vi "Table.Clear.vi"(8 "error in (no error)":errorcluster, 11 "State Variables":T1) -> (0 "error out":errorcluster)   [LabVIEW 2015]
uses:
  Types/Main.StateVariables.ctl
  <vilib>/Utility/miscctls.llb/LVPositionTypeDef.ctl
  Types/Execute.UserEventRefs.ctl
  <vilib>/NI Veristand/Execution/Workspace/SystemStateRegEventRef.ctl
  <vilib>/NI Veristand/Execution/Workspace/Target State Info.ctl
  <vilib>/NI Veristand/Execution/Workspace/Target State.ctl
  <vilib>/NI Veristand/Execution/WaveformStreaming/Waveform Data Watcher Event Data (DBL).ctl
  <vilib>/NI Veristand/Execution/WaveformStreaming/WaveformStreamSpecification.ctl
  NationalInstruments.VeriStand.ClientAPI
  <vilib>/NI Veristand/Execution/Workspace/SystemStateEventRef.ctl
  <vilib>/NI Veristand/Execution/Workspace/WorkspaceAPI.ctl
  Types/UI.Object.ctl
  Types/Waveforms.Info.ctl
  <vilib>/NI Veristand/Execution/WaveformStreaming/Registered Waveform Streams Data Event Refnum (DBL).ctl
  <vilib>/NI Veristand/Execution/WaveformStreaming/WaveformDataWatcherDBL.ctl
  <vilib>/NI Veristand/Execution/WaveformStreaming/WaveformStreamingAPI.ctl
  <vilib>/Utility/miscctls.llb/LVRowAndColumnTypeDef.ctl
  <vilib>/NI Veristand/Execution/Workspace/NI_VS Workspace ExecutionAPI.lvlib
  <vilib>/NI Veristand/Execution/WaveformStreaming/NI_VS Waveform Streaming Interface.lvlib
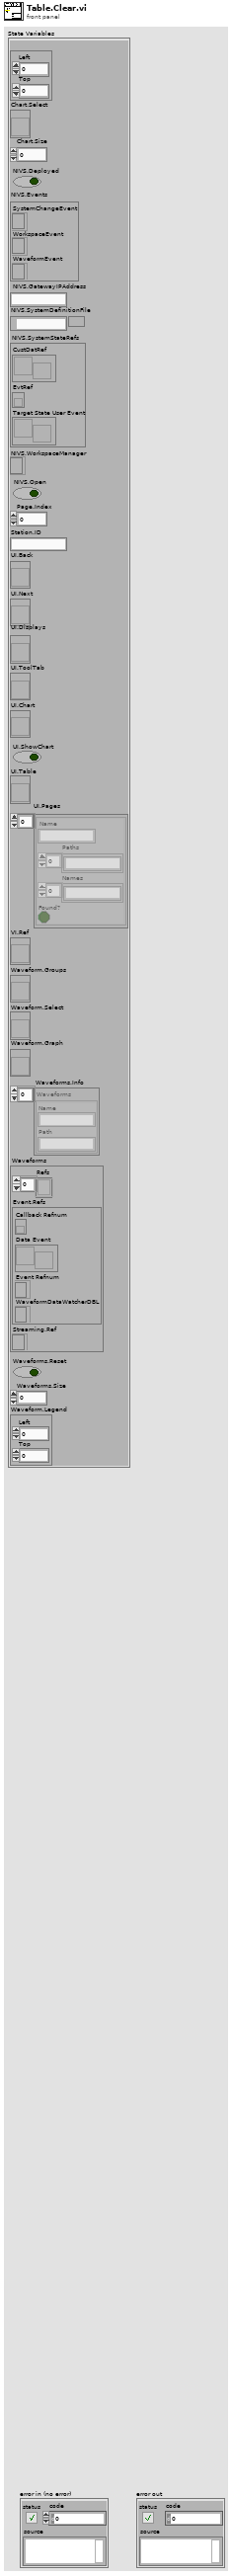
[diagram p1: front panel]
types:
  T1 = typedef "Main.StateVariables.ctl" = cluster{"Chart.Legend":T2, "Chart.Select":refnum<vi>, "Chart.Size":i32, "NIVS.Deployed":bool, "NIVS.Events":T3, "NIVS.GatewayIPAddress":string, "NIVS.SystemDefinitionFile":path, "NIVS.SystemStateRefs":T5, "NIVS.WorkspaceManager":T6, "NIVS.Open":bool, "Page.Index":u32, "Station.ID":string, "UI.Back":refnum<vi>, "UI.Next":refnum<vi>, "UI.Displays":refnum<vi>, "UI.ToolTab":refnum<vi>, "UI.Chart":refnum<vi>, "UI.ShowChart":bool, "UI.Table":refnum<vi>, "UI.Pages":T7[], "VI.Ref":refnum<vi>, "Waveform.Groups":refnum<vi>, "Waveform.Select":refnum<vi>, "Waveform.Graph":refnum<vi>, "Waveforms.Info":T8[], "Waveforms":cluster{"Refs":T9[], "Event.Refs":T10, "Streaming.Ref":T12}, "Waveforms.Reset":bool, "Waveforms.Size":i32, "Waveform.Legend":T2}
  T2 = typedef "LVPositionTypeDef.ctl" = cluster{"Left":i32, "Top":i32}
  T3 = typedef "Execute.UserEventRefs.ctl" = cluster{"SystemChangeEvent":T4, "WorkspaceEvent":refnum<event-registration>, "WaveformEvent":refnum<event-registration>}
  T4 = typedef "NI_VS Workspace ExecutionAPI.lvlib/SystemStateRegEventRef.ctl" = refnum<event-registration>
  T5 = typedef "NI_VS Workspace ExecutionAPI.lvlib/SystemStateEventRef.ctl" = cluster{"CustDatRef":refnum<user-event>, "EvtRef":refnum<k27>, "Target State User Event":refnum<user-event>}
  T6 = typedef "NI_VS Workspace ExecutionAPI.lvlib/WorkspaceAPI.ctl" = refnum<k24>
  T7 = typedef "UI.Object.ctl" = cluster{"Name":string, "Paths":string[], "Names":string[], "Found?":bool}
  T8 = typedef "Waveforms.Info.ctl" = cluster{"Name":string, "Path":string}
  T9 = typedef "NI_VS Waveform Streaming Interface.lvlib/WaveformStreamSpecification.ctl" = refnum<k24>
  T10 = typedef "NI_VS Waveform Streaming Interface.lvlib/Registered Waveform Streams Data Event Refnum (DBL).ctl" = cluster{"Callback Refnum":refnum<k27>, "Data Event":refnum<user-event>, "Event Refnum":refnum<event-registration>, "WaveformDataWatcherDBL":T11}
  T11 = typedef "NI_VS Waveform Streaming Interface.lvlib/WaveformDataWatcherDBL.ctl" = refnum<k24>
  T12 = typedef "NI_VS Waveform Streaming Interface.lvlib/WaveformStreamingAPI.ctl" = refnum<k24>
  T13 = typedef "LVRowAndColumnTypeDef.ctl" = cluster{"Row":i32, "Column":i32}
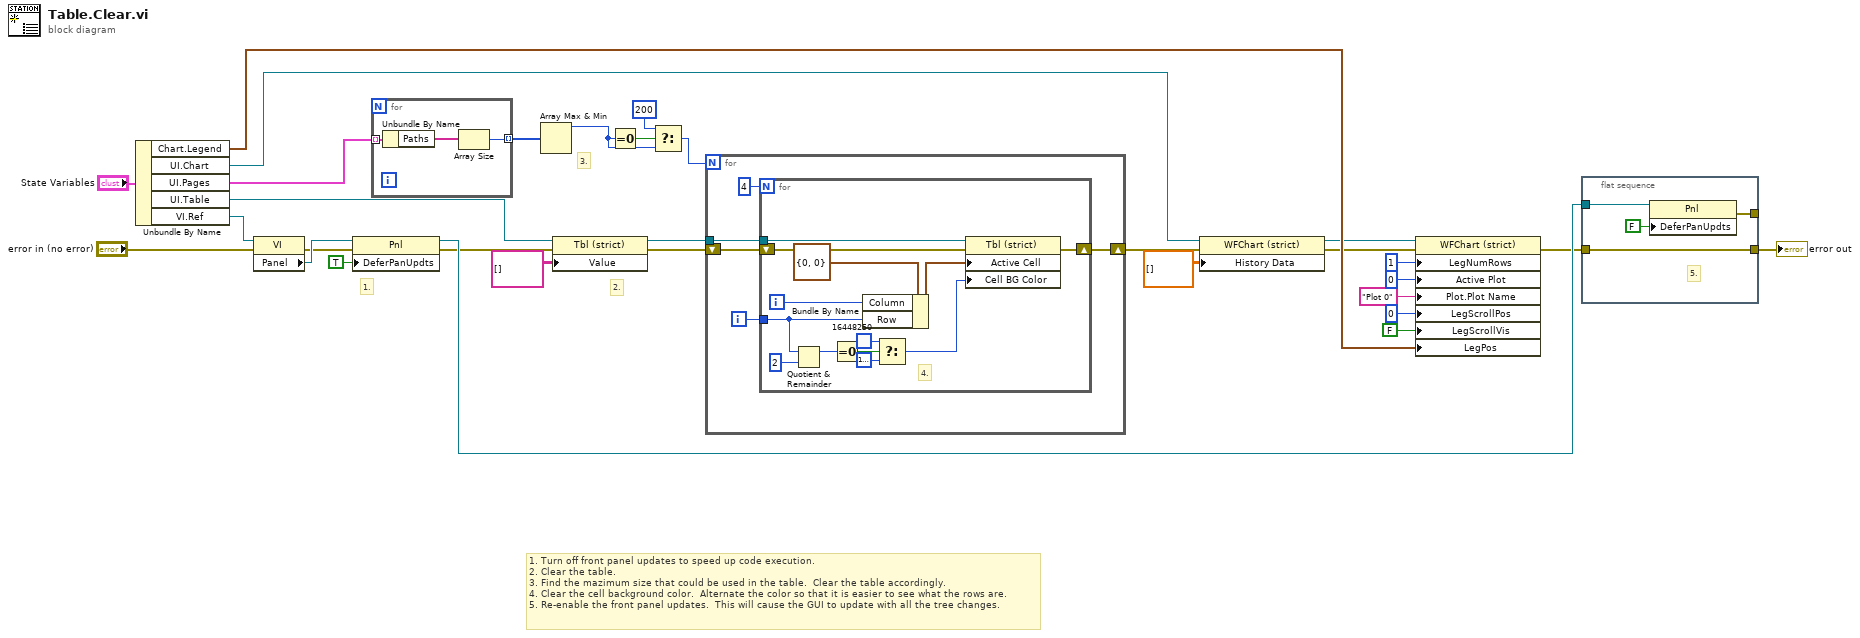
[diagram p0: block diagram]
diagram:
  # "3."
  # "2."
  # "1."
  # "1. Turn off front panel updates to speed up code execution.\n2. Clear the table.\n3. Find the mazimum size that could be used in the table.  Clear the table accordingly.\n4. Clear the cell background color.  Alternate the color so that it is easier to see what the rows are.\n5. Re-enable the front panel updates.  This will cause the GUI to update with all the tree changes."
  n1 = Unbundle By Name("State Variables") -> ("Chart.Legend"=w10:T2, "UI.Chart"=w13:refnum<vi>, "UI.Pages"=w24:T7[], "UI.Table"=w15:refnum<vi>, "VI.Ref"=w30:refnum<vi>)
  n2 = property class="VI"(reference=w30, error in="error in (no error)") -> (error out=w28:errorcluster, "Panel"=w29:refnum<vi>)  [unwired: 1 out]
  n3 = property class="Pnl"(reference=w29, error in=w28, "DeferPanUpdts"=TRUE ("Defer Panel Updates")) -> (reference out=w26:refnum<vi>, error out=w14:errorcluster)
  n4 = for {
    tunnel: w24 -> [w34] mode=indexing
    tunnel: [w32] -> w23 mode=indexing
    n5 = Unbundle By Name(w34) -> ("Paths"=w33:string[])
    n6 = Array Size(array=w33) -> (size(s)=w32:i32)
  }
  n7 = Array Max & Min(array=w23) -> (max value=w22:i32)  [unwired: 3 out]
  n8 = property class="Tbl (strict)"(reference=w15, error in=w14, "Value"=string[][] []) -> (reference out=w19:refnum<vi>, error out=w20:errorcluster)
  n9 = Equal To 0?(x=w22) -> (x = 0?=w18:bool)
  n10 = Select(t=200, s=w18, f=w22) -> (s? t:f=w16:i32)
  n11 = for {
    N: w16 -> [_]
    tunnel: w19 -> [w37]
    shift-right: [w38] -> w12
    shift-left: w20 -> [w39]
    i -> [w36]
    n12 = for {
      N: 4 -> [_]
      tunnel: w37 -> [w50]
      shift-right: [w51] -> w38
      shift-left: w39 -> [w52]
      tunnel: w36 -> [w47]
      i -> [w40]
      # "4."
      n13 = Quotient & Remainder(x=w47, y=2) -> (x-y*floor(x/y)=w45:i32)  [unwired: 1 out]
      n14 = Equal To 0?(x=w45) -> (x = 0?=w44:bool)
      n15 = Bundle By Name(cluster=T13 {"Row"=0, "Column"=0} ("Active Cell:Active Cell"), "Column"=w40, "Row"=w47) -> (w48:T13)
      n16 = Select(t=u32 16448250, s=w44, f=u32 16777238) -> (s? t:f=w41:u32)
      n17 = property class="Tbl (strict)"(reference=w50, error in=w52, "Active Cell"=w48, "Cell BG Color"=w41) -> (error out=w51:errorcluster)  [unwired: 1 out]
    }
  }
  n18 = property class="WFChart (strict)"(reference=w13, error in=w12, "History Data"=dbl[][] []) -> (reference out=w3:refnum<vi>, error out=w2:errorcluster)
  n19 = property class="WFChart (strict)"(reference=w3, error in=w2, "LegNumRows"=u32 1 ("Legend:Number of Rows"), "Active Plot"=u32 0, "Plot.Plot Name"="Plot 0", "LegScrollPos"=u32 0 ("Legend:Scroll Position"), "LegScrollVis"=FALSE ("Legend:Scrollbar Visible"), "LegPos"=w10) -> (error out=w11:errorcluster)  [unwired: 1 out]
  n20 = flat-sequence {
    tunnel: w26 -> [w56]
    tunnel: [w55] -> w25
    tunnel: w11 -> [w55]
    tunnel: [w54] -> _
    frame #0 {
      # "5."
      n21 = property class="Pnl"(reference=w56, "DeferPanUpdts"=FALSE ("Defer Panel Updates")) -> (error out=w54:errorcluster)  [unwired: 1 in, 1 out]
    }
  }
  "error out" <- w25
